vi "Configure Multi Eval Meas Modulation Results Enabled.vi"(7 "Enabled (Off)":bool, 8 "error in (no error)":errorcluster, 9 "Modulation (EVM)":i32(ring) items=["EVM", "EVM vs Subcarrier", "Magnitude Error", "Phase Error", "Inband Emissions", "IQ", "Equalizer Spectrum Flatness", "TX Measurement", "SEM", "ACLR"], 10 "Instance (1)":T1=1, 11 "VISA resource name":refnum<visa-resource-name>) -> (0 "error out":errorcluster, 3 "VISA resource name out":refnum<visa-resource-name>)   [LabVIEW 2020, in "Rohde&Schwarz CMWXP NR FR1 Measurement.lvlib"]
doc: "Enables or disables the evaluation of results in the multi-evaluation measurement.\n\nAttributes:\nRSCMWXPNRFR1M_ATTR_MULTI_EVAL_MEAS_MODULATION_EVM_RESULT_ENABLED\nRSCMWXPNRFR1M_ATTR_MULTI_EVAL_MEAS_MODULATION_EVMC_RESULT_ENABLED\nRSCMWXPNRFR1M_ATTR_MULTI_EVAL_MEAS_MODULATION_MAGNITUDE_ERROR_RESULT_ENABLED\nRSCMWXPNRFR1M_ATTR_MULTI_EVAL_MEAS_MODULATION_PHASE_ERROR_RESULT_ENABLED\nRSCMWXPNRFR1M_ATTR_MULTI_EVAL_MEAS_MODULATION_INBAND_EMISSIONS_RESULT_ENABLED\nRSCMWXPNRFR1M_ATTR_MULTI_EVAL_MEAS_MODULATION_IQ_RESULT_ENABLED\nRSCMWXPNRFR1M_ATTR_MULTI_EVAL_MEAS_MODULATION_EQ_SPECTRUM_FLATNESS_RESULT_ENABLED\nRSCMWXPNRFR1M_ATTR_MULTI_EVAL_MEAS_MODULATION_TX_MEASUREMENT_RESULT_ENABLED\nRSCMWXPNRFR1M_ATTR_MULTI_EVAL_MEAS_MODULATION_SEM_RESULT_ENABLED\nRSCMWXPNRFR1M_ATTR_MULTI_EVAL_MEAS_MODULATION_ACLR_RESULT_ENABLED\n\nRemote-control commands:\nCONFigure:NRSub:MEAS<i>:MEValuation:RESult:EVMagnitude\nCONFigure:NRSub:MEAS<i>:MEValuation:RESult:EVMC\nCONFigure:NRSub:MEAS<i>:MEValuation:RESult:MERRor\nCONFigure:NRSub:MEAS<i>:MEValuation:RESult:PERRor\nCONFigure:NRSub:MEAS<i>:MEValuation:RESult:IEMissions\nCONFigure:NRSub:MEAS<i>:MEValuation:RESult:IQ\nCONFigure:NRSub:MEAS<i>:MEValuation:RESult:ESFLatness\nCONFigure:NRSub:MEAS<i>:MEValuation:RESult:TXM\nCONFigure:NRSub:MEAS<i>:MEValuation:RESult:SEMask\nCONFigure:NRSub:MEAS<i>:MEValuation:RESult:ACLR"
uses:
  <instrlib>/Rohde&Schwarz CMWXP NR FR1 Measurement/Rohde&Schwarz CMWXP NR FR1 Measurement.lvlib
  <instrlib>/Rohde&Schwarz CMWXP NR FR1 Measurement/Private/_Instance.ctl
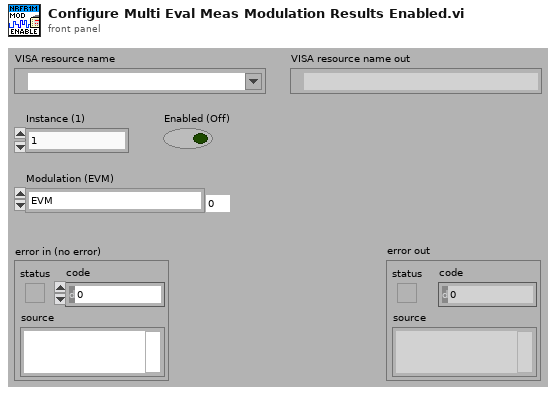
[diagram p1: front panel]
types:
  T1 = typedef "Rohde&Schwarz CMWXP NR FR1 Measurement.lvlib/_Instance.ctl" = i32
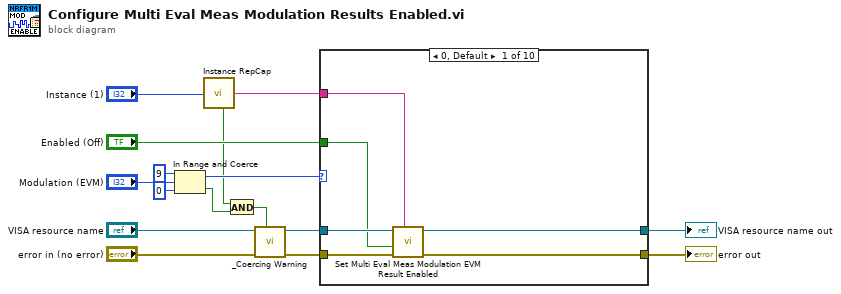
[diagram p0: block diagram]
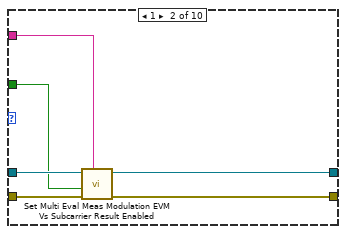
[diagram p2: hidden frame]
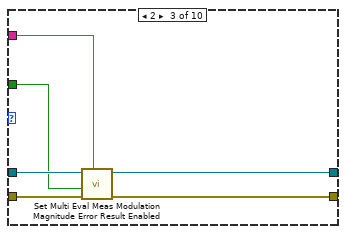
[diagram p3: hidden frame]
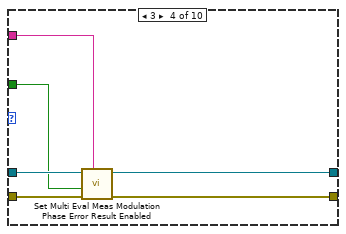
[diagram p4: hidden frame]
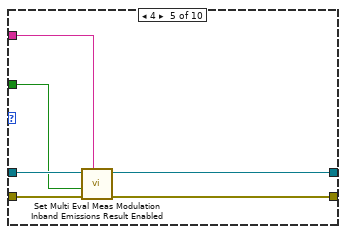
[diagram p5: hidden frame]
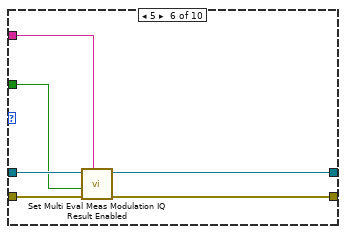
[diagram p6: hidden frame]
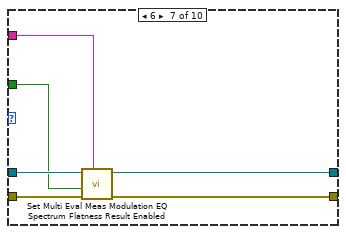
[diagram p7: hidden frame]
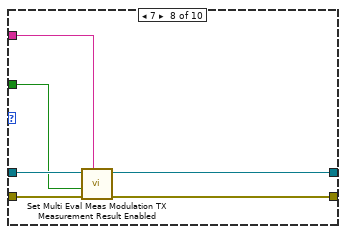
[diagram p8: hidden frame]
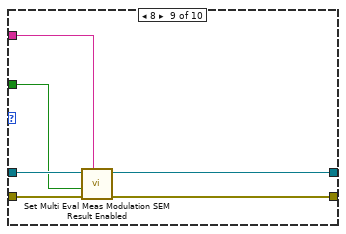
[diagram p9: hidden frame]
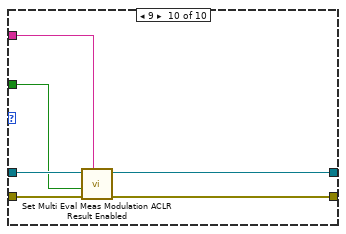
[diagram p10: hidden frame]
diagram:
  n1 = In Range and Coerce(upper limit=9, x="Modulation (EVM)", lower limit=0) -> (coerced(x)=w6:i32, In Range?=w2:bool)
  n2 = call <instrlib>:"Instance RepCap.vi"("Instance In"="Instance (1)") -> ("In Range?"=w1:bool, "RepCap Identifier Out"=w13:string)  [unwired: 1 in]
  n3 = And(x=w1, y=w2) -> (x .and. y?=w3:bool)
  n4 = call <instrlib>:"_Coercing Warning.vi"("In Range?"=w3, "error in (no error)"="error in (no error)", "VISA resource name"="VISA resource name") -> ("error out"=w9:errorcluster, "VISA resource name out"=w8:refnum<visa-resource-name>)  [unwired: 7 in]
  n5 = case shown="0, Default" w6 {
    tunnel: w9 -> [w22 w28 w34 w40 w46 w52 w58 w64 w70 w76]
    tunnel: [w21 w27 w33 w39 w45 w51 w57 w63 w69 w75] -> w16
    tunnel: w8 -> [w20 w26 w32 w38 w44 w50 w56 w62 w68 w74]
    tunnel: [w19 w25 w31 w37 w43 w49 w55 w61 w67 w73] -> w15
    tunnel: w13 -> [w18 w24 w30 w36 w42 w48 w54 w60 w66 w72]
    tunnel: "Enabled (Off)" -> [w17 w23 w29 w35 w41 w47 w53 w59 w65 w71]
    frame 0, Default {
      n6 = call "Set Multi Eval Meas Modulation EVM Result Enabled"("Repeated Capabilities"=w18, "error in (no error)"=w22, "Multi Eval Meas Modulation EVM Result Enabled (OFF)"=w17, "instrument handle"=w20) -> ("error out"=w21:errorcluster, "instrument handle out"=w19:refnum<visa-resource-name>)  [unwired: 6 in]
    }
    frame 1 {
      n7 = call "Set Multi Eval Meas Modulation EVM Vs Subcarrier Result Enabled"("Repeated Capabilities"=w24, "error in (no error)"=w28, "Multi Eval Meas Modulation EVM Vs Subcarrier Result Enabled (OFF)"=w23, "instrument handle"=w26) -> ("error out"=w27:errorcluster, "instrument handle out"=w25:refnum<visa-resource-name>)  [unwired: 6 in]
    }
    frame 2 {
      n8 = call "Set Multi Eval Meas Modulation Magnitude Error Result Enabled"("Repeated Capabilities"=w30, "error in (no error)"=w34, "Multi Eval Meas Modulation Magnitude Error Result Enabled (OFF)"=w29, "instrument handle"=w32) -> ("error out"=w33:errorcluster, "instrument handle out"=w31:refnum<visa-resource-name>)  [unwired: 6 in]
    }
    frame 3 {
      n9 = call "Set Multi Eval Meas Modulation Phase Error Result Enabled"("Repeated Capabilities"=w36, "error in (no error)"=w40, "Multi Eval Meas Modulation Phase Error Result Enabled (OFF)"=w35, "instrument handle"=w38) -> ("error out"=w39:errorcluster, "instrument handle out"=w37:refnum<visa-resource-name>)  [unwired: 6 in]
    }
    frame 4 {
      n10 = call "Set Multi Eval Meas Modulation Inband Emissions Result Enabled"("Repeated Capabilities"=w42, "error in (no error)"=w46, "Multi Eval Meas Modulation Inband Emissions Result Enabled (OFF)"=w41, "instrument handle"=w44) -> ("error out"=w45:errorcluster, "instrument handle out"=w43:refnum<visa-resource-name>)  [unwired: 6 in]
    }
    frame 5 {
      n11 = call "Set Multi Eval Meas Modulation IQ Result Enabled"("Repeated Capabilities"=w48, "error in (no error)"=w52, "Multi Eval Meas Modulation IQ Result Enabled (OFF)"=w47, "instrument handle"=w50) -> ("error out"=w51:errorcluster, "instrument handle out"=w49:refnum<visa-resource-name>)  [unwired: 6 in]
    }
    frame 6 {
      n12 = call "Set Multi Eval Meas Modulation EQ Spectrum Flatness Result Enabled"("Repeated Capabilities"=w54, "error in (no error)"=w58, "Multi Eval Meas Modulation EQ Spectrum Flatness Result Enabled (OFF)"=w53, "instrument handle"=w56) -> ("error out"=w57:errorcluster, "instrument handle out"=w55:refnum<visa-resource-name>)  [unwired: 6 in]
    }
    frame 7 {
      n13 = call "Set Multi Eval Meas Modulation TX Measurement Result Enabled"("Repeated Capabilities"=w60, "error in (no error)"=w64, "Multi Eval Meas Modulation TX Measurement Result Enabled (OFF)"=w59, "instrument handle"=w62) -> ("error out"=w63:errorcluster, "instrument handle out"=w61:refnum<visa-resource-name>)  [unwired: 6 in]
    }
    frame 8 {
      n14 = call "Set Multi Eval Meas Modulation SEM Result Enabled"("Repeated Capabilities"=w66, "error in (no error)"=w70, "Multi Eval Meas Modulation SEM Result Enabled (OFF)"=w65, "instrument handle"=w68) -> ("error out"=w69:errorcluster, "instrument handle out"=w67:refnum<visa-resource-name>)  [unwired: 6 in]
    }
    frame 9 {
      n15 = call "Set Multi Eval Meas Modulation ACLR Result Enabled"("Repeated Capabilities"=w72, "error in (no error)"=w76, "Multi Eval Meas Modulation ACLR Result Enabled (OFF)"=w71, "instrument handle"=w74) -> ("error out"=w75:errorcluster, "instrument handle out"=w73:refnum<visa-resource-name>)  [unwired: 6 in]
    }
  }
  "error out" <- w16
  "VISA resource name out" <- w15
